vi "Execute.vi"(8 "error in (no error)":errorcluster, 11 "UDP_Comm in":refnum<class "UDP_Comm.lvclass">) -> (0 "error out":errorcluster, 3 "UDP_Comm out":refnum<class "UDP_Comm.lvclass">)   [LabVIEW 2021, in "UDP_Comm.lvclass"]
uses:
  UDP_Comm.lvclass
  UDP_Comm.lvclass/UDP_Comm.ctl
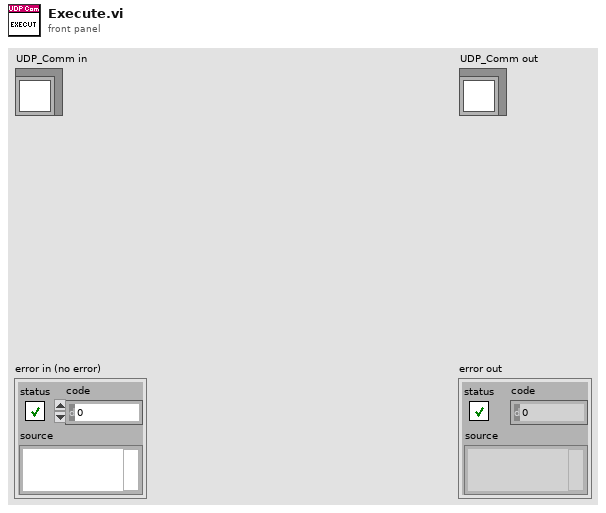
[diagram p1: front panel]
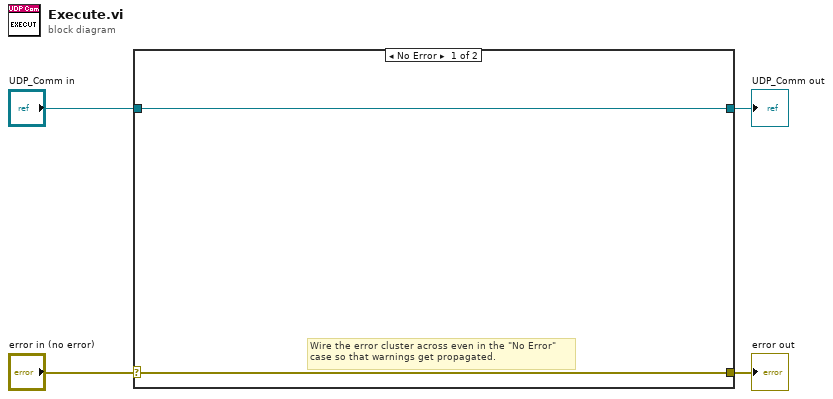
[diagram p0: block diagram]
diagram:
  n1 = case shown="No Error" "error in (no error)" {
    selector: "error in (no error)" -> [w5 w8]
    tunnel: [w5 w8] -> w3
    tunnel: [w6 w7] -> w1
    tunnel: "UDP_Comm in" -> [w6 w7]
    frame No Error {
      # "Wire the error cluster across even in the \"No Error\"\ncase so that warnings get propagated."
    }
    frame Error {
    }
  }
  "error out" <- w3
  "UDP_Comm out" <- w1
